vi "Set Port Name by Config.vi"(10 "Redundant?":bool, 11 "port id":i32) -> (3 "Port name out":string)   [LabVIEW 2020, in "AIM ARINC 664 Scripting.lvlib"]
uses:
  AIM ARINC 664 Scripting.lvlib
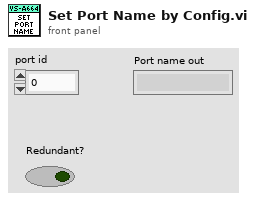
[diagram p1: front panel]
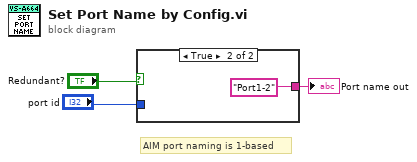
[diagram p0: block diagram]
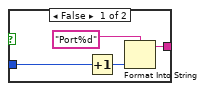
[diagram p2: hidden frame]
diagram:
  # "AIM port naming is 1-based"
  n1 = case shown="True" "Redundant?" {
    tunnel: [w7 "Port1-2"] -> w2
    tunnel: "port id" -> [w4 _]
    frame False {
      n2 = Increment(x=w4) -> (x+1=w5:i32)
      n3 = Format Into String(format string="Port%d", w5) -> (resulting string=w7:string)  [unwired: 2 in, 1 out]
    }
    frame True {
    }
  }
  "Port name out" <- w2
